vi "Read Single Analog.vi"(0 "Device ID":T3(ring), 5 "Module":T2(ring), 7 "Analog_Input":T1(ring)=enum."Input A1", 11 "error in":errorcluster) -> (4 "Device ID Out":T3(ring), 6 "Value":u16, 15 "error out":errorcluster)   [LabVIEW 2010]
doc: "This VI reads a single analog input from the transfer area."
uses:
  Robo Interface.dll
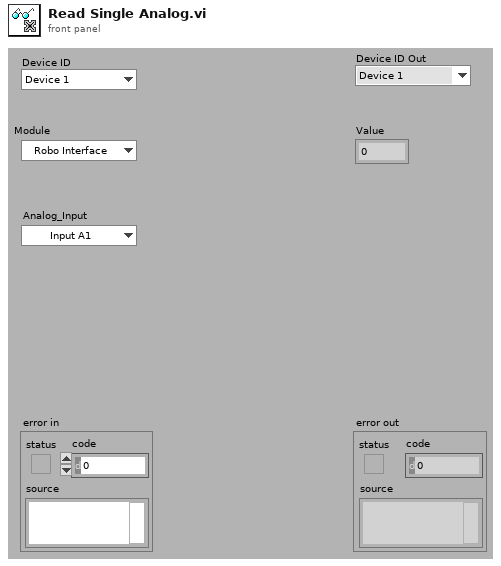
[diagram p1: front panel]
types:
  T1 = enum8{"Input AX", "Input AY", "Input A1", "Input A2", "Input AZ", "Input AV", "Input D1", "Input D2", "Input AXR", "Input AYR"}
  T2 = enum8{"Robo Interface", "Extension 1", "Extension 2", "Extension 3"}
  T3 = enum16{"Device 1", "Device 2", "Device 3", "Device 4", "Device 5", "Device 6", "Device 7", "Device 8"}
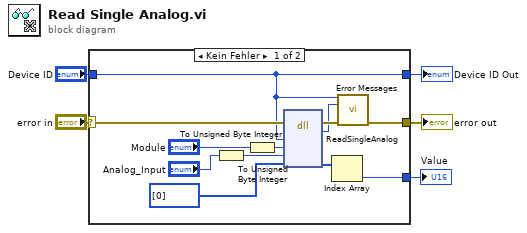
[diagram p0: block diagram]
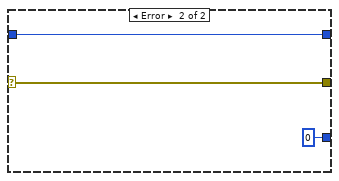
[diagram p2: hidden frame]
diagram:
  n1 = case shown="Kein Fehler" "error in" {
    selector: "error in" -> [w14 w20]
    tunnel: [w12 w20] -> w4
    tunnel: "Device ID" -> [w6 w19]
    tunnel: [w6 w19] -> w2
    tunnel: [w8 u16 0] -> w1
    frame No Error {
      n2 = To Unsigned Byte Integer(number="Analog_Input") -> (unsigned 8bit integer=w10:u8)
      n3 = To Unsigned Byte Integer(number="Module") -> (unsigned 8bit integer=w11:u8)
      n4 = dll-call lib="D:/Aron/LabVIEW-Programmierung/a.F.b.u.s.A/robo_interface_distribute/Robo Interface/Advanced/Robo Interface.dll" fn="ReadSingleAnalog"(error in=w14, "Device_ID"=w6, "Module"=w11, "Type"=w10, "Value"=u16[] [0]) -> (error out=w13:errorcluster, "return type"=w7:i32, "Value"=w9:u16[])  [unwired: 4 in, 2 out]
      n5 = Index Array(array=w9) -> (element=w8:u16)  [unwired: 1 in]
      n6 = call "Error Messages.vi"("Device ID"=w6, "Error Code"=w7, "error in (no error)"=w13) -> ("error out"=w12:errorcluster)  [unwired: 12 out]
    }
    frame Error {
    }
  }
  "error out" <- w4
  "Device ID Out" <- w2
  "Value" <- w1
